vi "mensagemvisor.vi"(0 "NXT IN":T1) -> (1 "NXT OUT":T1, 2 "FinalizarPrograma?":bool)   [LabVIEW 2015, in "ExemploFinal.lvrbt"]
uses:
  ExemploFinal.lvrbt
  <vilib>/NXT/Subs/LVHSConnector.ctl
  <vilib>/NXT/LegoClasses/BrickReference/BrickReference.lvclass
  <vilib>/NXT/Dual Mode Library/Display/clearDisplay.vi
  <vilib>/NXT/Dual Mode Library/Display/drawText_Center.vi
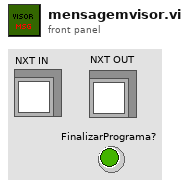
[diagram p1: front panel]
types:
  T1 = typedef "LVHSConnector.ctl" = refnum<class "BrickReference.lvclass">
  T2 = cluster{"MSG_TouchOUT":string, "MSG_SomOUT":string, "MSG_LuzOUT":string, "MSG_UltrasomOUT":string, "MSG_BotãoOUT":string}
  T3 = cluster{"TouchOUT":bool, "SomOUT":i32, "LuzOUT":i32, "UltrasomOUT":i32, "BotãoOUT":bool}
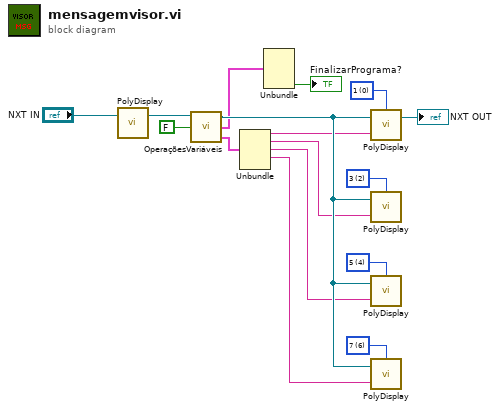
[diagram p0: block diagram]
diagram:
  w14 = i16 6 items=["1", "2", "3", "4", "5", "6", "7", "8", "9", "10", "11", "12"] ("Line")
  w15 = i16 4 items=["1", "2", "3", "4", "5", "6", "7", "8", "9", "10", "11", "12"] ("Line")
  w13 = i16 2 items=["1", "2", "3", "4", "5", "6", "7", "8", "9", "10", "11", "12"] ("Line")
  w12 = i16 0 items=["1", "2", "3", "4", "5", "6", "7", "8", "9", "10", "11", "12"] ("Line")
  n1 = call-poly <vilib>:"PolyDisplay.vi"("NXT/EV3"="NXT IN") -> ("NXT/EV3"=w11:T1)  [unwired: 3 in]
  n2 = call "OperaçõesVariáveis.vi"("Escrever?"=FALSE, "NXT IN"=w11) -> ("Mensagens"=w7:T2, "Saídas"=w2:T3, "NXT OUT"=w8:T1)  [unwired: 1 in]
  n3 = Unbundle(w7) -> ("MSG_TouchOUT"=w6:string, "MSG_SomOUT"=w5:string, "MSG_LuzOUT"=w4:string, "MSG_UltrasomOUT"=w3:string)  [unwired: 1 out]
  n4 = Unbundle(w2) -> ("BotãoOUT"=→"FinalizarPrograma?":bool)  [unwired: 4 out]
  n5 = call-poly <vilib>:"PolyDisplay.vi"("Text"=w6, "NXT/EV3"=w8, "Line"=w12) -> ("NXT/EV3"=→"NXT OUT":T1)  [unwired: 1 in]
  n6 = call-poly <vilib>:"PolyDisplay.vi"("Text"=w5, "NXT/EV3"=w8, "Line"=w13) -> ()  [unwired: 1 in, 1 out]
  n7 = call-poly <vilib>:"PolyDisplay.vi"("Text"=w4, "NXT/EV3"=w8, "Line"=w15) -> ()  [unwired: 1 in, 1 out]
  n8 = call-poly <vilib>:"PolyDisplay.vi"("Text"=w3, "NXT/EV3"=w8, "Line"=w14) -> ()  [unwired: 1 in, 1 out]
